vi "Parse Transfer Group.vi"(8 "error in (no error)":errorcluster, 10 "Transfer Group in":refnum<class "Transfer Group.lvclass">, 11 "Plugin Thread in":refnum<class "Transceiver Thread.lvclass">) -> (0 "error out":errorcluster, 2 "Transfer Group out":refnum<class "Transfer Group.lvclass">, 3 "Plugin Thread out":refnum<class "Transceiver Thread.lvclass">)   [LabVIEW 2019, in "DSF Core.lvlib" / "Transceiver Thread.lvclass"]
uses:
  Transceiver Thread.lvclass
  Transfer Group/Transfer Group.lvclass
  Transceiver Thread.lvclass/Transceiver Thread.ctl
  Buffer Converter/Buffer Converter.lvclass
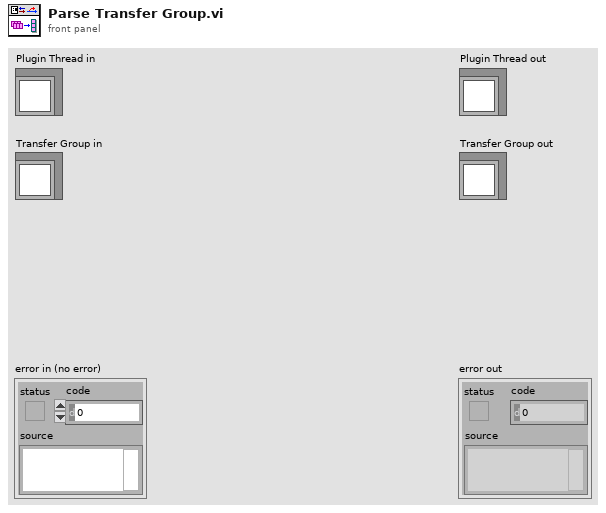
[diagram p1: front panel]
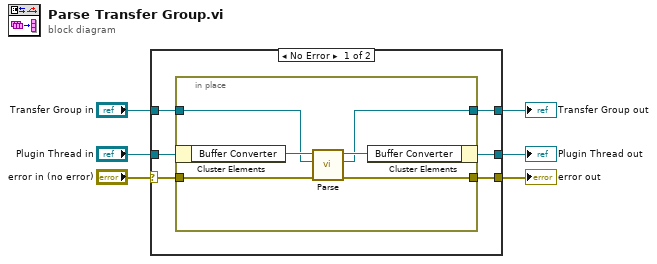
[diagram p0: block diagram]
diagram:
  n1 = case shown="No Error" "error in (no error)" {
    selector: "error in (no error)" -> [w7 w19]
    tunnel: [w12 w19] -> w6
    tunnel: [w11 w20] -> w5
    tunnel: "Plugin Thread in" -> [w10 w20]
    tunnel: "Transfer Group in" -> [w9 w21]
    tunnel: [w8 w21] -> w2
    frame No Error {
      n2 = in-place {
        in-place-border: w7 -> [w16]
        in-place-border: [w15] -> w12
        in-place-border: w9 -> [w14]
        in-place-border: [w13] -> w8
        n3 = in-place-cluster #1(w10) -> ("Buffer Converter"=w18:refnum<class "Buffer Converter.lvclass">)
        n4 = call-dynamic "Parse.vi"("error in (no error)"=w16, "Transfer Group in"=w14, "Buffer Converter in"=w18) -> ("error out"=w15:errorcluster, "Transfer Group out"=w13:refnum<class "Transfer Group.lvclass">, "Buffer Converter out"=w17:refnum<class "Buffer Converter.lvclass">)  [unwired: 6 in]
        n5 = in-place-cluster #1("Buffer Converter"=w17) -> (w11:refnum<class "Transceiver Thread.lvclass">)
      }
    }
    frame Error {
    }
  }
  "error out" <- w6
  "Plugin Thread out" <- w5
  "Transfer Group out" <- w2
